vi "OneSessOnePinOneInstrTwoSitesReservation_CallGetConnectionsFromPinForOnePinAllSites_ReturnsTwoConnections.vi"(8 "error in":errorcluster) -> (0 "error out":errorcluster, 2 "result":string, 3 "pass":bool)   [LabVIEW 2020, in "MeasurementServerTests.lvlib"]
uses:
  MeasurementServerTests.lvlib
  Runtime/MeasurementLink Session Management/Session Reservation/Connection.ctl
  Runtime/MeasurementLink Session Management/Session Reservation/Hardware Independent Connection.ctl
  977fab1f-3164-461c-a2e7-4456bbbe5203.vi
  b3e5c3be-b7a7-4b6e-86ee-709eea9cb752.vi
  977fab1f-3164-461c-a2e7-4456bbbe5203.vi/10aac40e-32b1-41e4-9263-c4508fa95940.vi
  Runtime/MeasurementLink Session Management/Session Reservation/Get Connections Impl.vi
  Runtime/MeasurementLink Session Management/Session Reservation/Session Reservation.lvclass
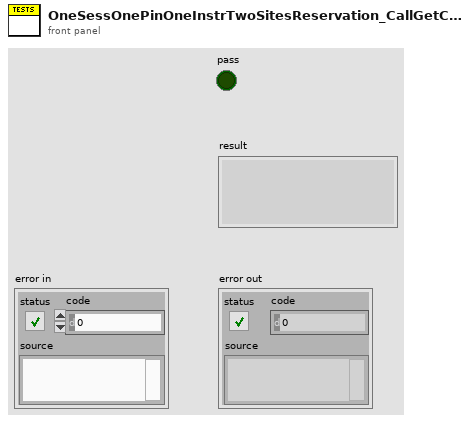
[diagram p1: front panel]
types:
  T1 = typedef "MeasurementLink Session Management.lvlib/Session Reservation.lvclass/Connection.ctl" = cluster{"connection":T2, "session":variant}
  T2 = typedef "MeasurementLink Session Management.lvlib/Session Reservation.lvclass/Hardware Independent Connection.ctl" = cluster{"pin or relay name":string, "site":i32, "instrument type id":string, "channel":string}
  T3 = typedef "MeasurementLink Session Management.lvlib/Session Reservation.lvclass/Data.ctl" = cluster{"session and driver infos":T4[], "pins":string[]}
  T4 = typedef "MeasurementLink Session Management.lvlib/Session Reservation.lvclass/Session and Driver Info.ctl" = cluster{"session info":T5, "session created":bool, "session":variant}
  T5 = typedef "MeasurementLink Session Management Client.lvlib/ni_measurementlink_sessionmanagement_v1_SessionInformation.ctl" = cluster{"session":T6, "resource_name":string, "channel_list":string, "instrument_type_id":string, "session_exists":bool, "channel_mappings":T7[]}
  T6 = typedef "MeasurementLink Session Management Client.lvlib/nidevice_grpc_Session.ctl" = cluster{"name":string}
  T7 = typedef "MeasurementLink Session Management Client.lvlib/ni_measurementlink_sessionmanagement_v1_ChannelMapping.ctl" = cluster{"pin_or_relay_name":string, "site":i32, "channel":string}
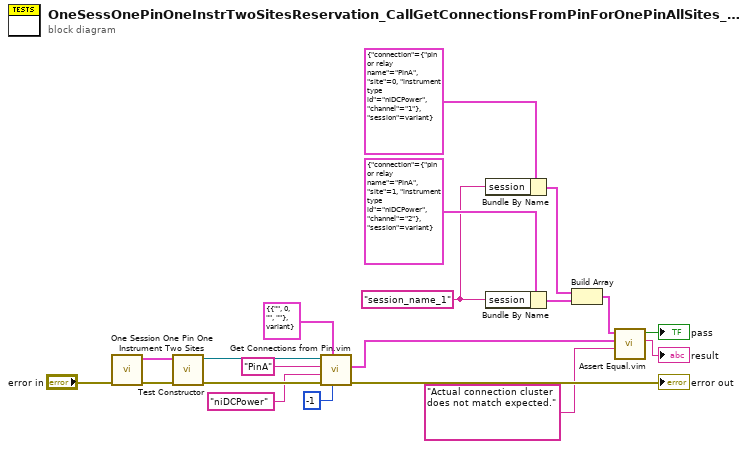
[diagram p0: block diagram]
diagram:
  w4 = "session_name_1"
  n1 = call "One Session One Pin One Instrument Two Sites.vi"("error in"="error in") -> ("error out"=w7:errorcluster, "data out"=w6:T3)  [unwired: 9 in]
  n2 = call "Test Constructor.vi"("error in"=w7, "data"=w6) -> ("error out"=w19:errorcluster, "Session Reservation out"=w18:refnum<class "Session Reservation.lvclass">)  [unwired: 8 in]
  n3 = call "Get Connections from Pin.vim"("site"=-1, "connection type"=T1 {"connection"={"pin or relay name"="", "site"=0, "instrument type id"="", "channel"=""}, "session"=variant} ("connection"), "error in"=w19, "instrument type id"="niDCPower", "pin or relay name"="PinA", "session reservation in"=w18) -> ("error out"=→"error out":errorcluster, "connections"=w16:T1[])  [unwired: 3 in, 1 out]
  n4 = Bundle By Name(cluster=T1 {"connection"={"pin or relay name"="PinA", "site"=0, "instrument type id"="niDCPower", "channel"="1"}, "session"=variant} ("connection"), "session"=w4) -> (w3:T1)
  n5 = Bundle By Name(cluster=T1 {"connection"={"pin or relay name"="PinA", "site"=1, "instrument type id"="niDCPower", "channel"="2"}, "session"=variant} ("connection"), "session"=w4) -> (w2:T1)
  n6 = Build Array(w3, w2) -> (w1:T1[])
  n7 = call "Assert Equal.vim"("failure message"="Actual connection cluster does not match expected.", "actual value"=w16, "expected value"=w1) -> ("message"=→"result":string, "equal?"=→"pass":bool)  [unwired: 7 in]
